vi "Set_Barometer_Calibration.vi"(2 "Elevation":i32, 3 "Sea level in":dbl, 4 "Path":path) -> (0 "Calibration values set?":bool, 1 "Barometer":dbl)   [LabVIEW 2012]
uses:
  <vilib>/Utility/config.llb/Write Key (Double).vi
  <vilib>/Utility/config.llb/Write Key (I32).vi
  VantagePro.dll
  <vilib>/Utility/config.llb/NI_LVConfig.lvlib
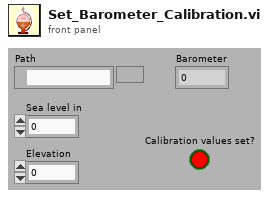
[diagram p1: front panel]
types:
  T1 = typedef "NI_LVConfig.lvlib/Config Data RefNum.ctl" = refnum<k1>
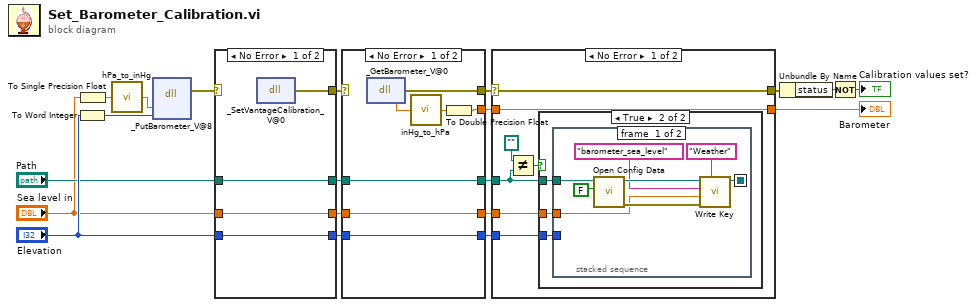
[diagram p0: block diagram]
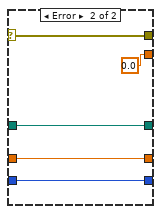
[diagram p2: hidden frame]
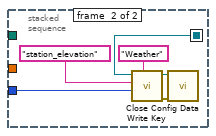
[diagram p4: hidden frame]
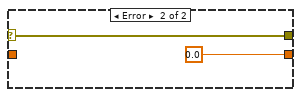
[diagram p5: hidden frame]
diagram:
  n1 = To Word Integer(number="Elevation") -> (16bit integer=w12:i16)
  n2 = To Single Precision Float(number="Sea level in") -> (single precision float=w8:sgl)
  n3 = call "hPa_to_inHg.vi"("hPa"=w8) -> ("inHg"=w17:sgl)
  n4 = dll-call lib="C:/Users/Bob van Eijk/Desktop/LabView Projects 12/HiSPARC Weather Station/Develop/VantagePro.dll" fn="_PutBarometer_V@8" label="Barometer value"("pressure"=w17, "elevation"=w12) -> (error out=w16:errorcluster)  [unwired: 6 in, 1 out]
  n5 = case shown="No Error" w16 {
    selector: w16 -> [_ w28]
    tunnel: [w24 w28] -> w19
    tunnel: "Elevation" -> [w23 w26]
    tunnel: [w23 w26] -> w11
    tunnel: "Sea level in" -> [w22 w27]
    tunnel: [w22 w27] -> w7
    tunnel: [w21 w25] -> w4
    tunnel: "Path" -> [w21 w25]
    frame No Error {
      n6 = dll-call lib="C:/Users/Bob van Eijk/Desktop/LabView Projects 12/HiSPARC Weather Station/Develop/VantagePro.dll" fn="_SetVantageCalibration_V@0" label="Set barometer values"() -> (error out=w24:errorcluster)  [unwired: 4 in, 1 out]
    }
    frame Error {
    }
  }
  n7 = case shown="No Error" w19 {
    selector: w19 -> [_ w40]
    tunnel: [w34 w40] -> w15
    tunnel: [w32 w38] -> w10
    tunnel: w11 -> [w32 w38]
    tunnel: w7 -> [w33 w39]
    tunnel: [w33 w39] -> w9
    tunnel: [w30 0.0] -> w2
    tunnel: [w29 w37] -> w5
    tunnel: w4 -> [w29 w37]
    frame No Error {
      n8 = dll-call lib="C:/Users/Bob van Eijk/Desktop/LabView Projects 12/HiSPARC Weather Station/Develop/VantagePro.dll" fn="_GetBarometer_V@0" label="Get Barometer"() -> (error out=w34:errorcluster, "return type"=w35:sgl)  [unwired: 3 in, 1 out]
      n9 = call "inHg_to_hPa.vi"("inHg"=w35) -> ("hPa"=w31:sgl)
      n10 = To Double Precision Float(number=w31) -> (double precision float=w30:dbl)
    }
    frame Error {
    }
  }
  n11 = case shown="No Error" w15 {
    selector: w15 -> [w45 w66]
    tunnel: w9 -> [w47 _]
    tunnel: w10 -> [w46 _]
    tunnel: [w45 w66] -> w14
    tunnel: w2 -> [w44 _]
    tunnel: [w44 0.0] -> w13
    tunnel: w5 -> [w41 _]
    frame No Error {
      n12 = Not Equal?(x=path "", y=w41) -> (x != y?=w42:bool)
      n13 = case shown="True" w42 {
        tunnel: w47 -> [_ w48]
        tunnel: w46 -> [_ w50]
        tunnel: w41 -> [_ w49]
        frame False {
        }
        frame True {
          n14 = stacked-sequence {
            seq-local: [w55 _] -> [_ w64]
            tunnel: w49 -> [w56 _]
            tunnel: w50 -> [_ w59]
            tunnel: w48 -> [w51 _]
            frame #0 {
              n15 = call <vilib>:"Open Config Data.vi"("create file if necessary (T)"=FALSE, "configuration file path"=w56) -> ("error out"=w52:errorcluster, "refnum"=w57:T1)  [unwired: 7 in, 1 out]
              n16 = call-poly <vilib>:"Write Key.vi"("section"="Weather" ("key"), "error in (no error)"=w52, "value"=w51, "key"="barometer_sea_level", "refnum"=w57) -> ("refnum out"=w55:T1)  [unwired: 4 in, 2 out]
            }
            frame #1 {
              n17 = call-poly <vilib>:"Write Key.vi"("section"="Weather" ("key"), "value"=w59, "key"="station_elevation", "refnum"=w64) -> ("error out"=w60:errorcluster, "refnum out"=w61:T1)  [unwired: 5 in, 1 out]
              n18 = call <vilib>:"Close Config Data.vi"("error in (no error)"=w60, "refnum"=w61) -> ()  [unwired: 8 in, 2 out]
            }
          }
        }
      }
    }
    frame Error {
    }
  }
  "Barometer" <- w13
  n19 = Unbundle By Name(w14) -> ("status"=w20:bool)
  n20 = Not(x=w20) -> (.not. x?=→"Calibration values set?":bool)
